vi "Calc.vi"(8 "error in (no error)":errorcluster, 10 "ArrayOfWVFMs":waveform(dbl)[](array[waveform]), 11 "AbstractCalc in":refnum<class "AbstractCalc.lvclass">) -> (0 "error out":errorcluster, 2 "Results":string[](array[string]), 3 "AbstractCalc out":refnum<class "AbstractCalc.lvclass">)   [LabVIEW 2015, in "AbstractCalcLib.lvlib" / "AbstractCalc.lvclass"]
uses:
  AbstractCalc.lvclass
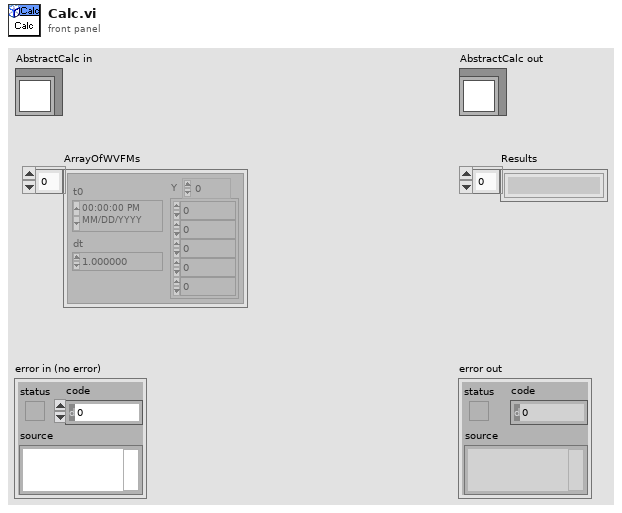
[diagram p1: front panel]
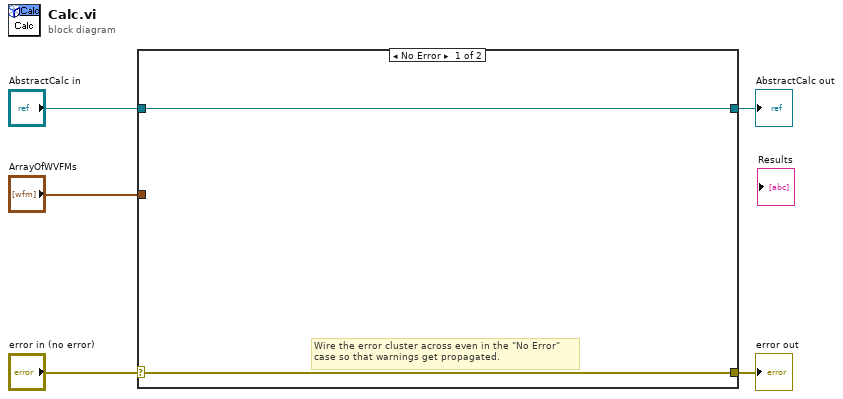
[diagram p0: block diagram]
diagram:
  n1 = case shown="No Error" "error in (no error)" {
    selector: "error in (no error)" -> [w6 w9]
    tunnel: [w6 w9] -> w4
    tunnel: [w7 w8] -> w2
    tunnel: "AbstractCalc in" -> [w7 w8]
    tunnel: "ArrayOfWVFMs" -> [_ _]
    frame No Error {
      # "Wire the error cluster across even in the \"No Error\"\ncase so that warnings get propagated."
    }
    frame Error {
    }
  }
  "error out" <- w4
  "AbstractCalc out" <- w2
